vi "06. Native MQTT System.vi"() -> ()   [LabVIEW 2019]
uses:
  Actor/Request -- cluster.ctl
  <vilib>/LabVIEW Open Source Project/MQTT Control Packets/Control Packets/ControlPacket/ControlPacket.lvclass/ControlPacket.ctl
  d83398bf-d288-4447-9c56-1851baa950d7.vi
  04c4b1fc-7be5-4a64-96c3-6608f790954d.vi
  6d0c06f0-3ef9-43f7-be9c-84012acbe03f.vi
  e0405e1f-2754-44b6-a86d-f374eef61912.vi
  <vilib>/LabVIEW Open Source Project/MQTT Control Packets/Control Packets/PUBLISH/PUBLISH.lvclass
  C:/Program Files (x86)/National Instruments/LabVIEW 2019/vi.lib/LabVIEW Open Source Project/MQTT Control Packets/Control Packets/ControlPacket/ControlPacket.lvclass
  <vilib>/JDP Science/JSONtext/JSON text to Variant.vi
  <vilib>/JDP Science/JSONtext/Variant to JSON Text.vi
  <vilib>/JDP Science/JSONtext/LVClass Serializer/JSONtext LVClass Serializer.lvclass
  <vilib>/LabVIEW Open Source Project/MQTT Control Packets/Control Packets/ControlPacket/ControlPacket.lvclass
panel:
  in  "QualifiedName":string="demo/system"
  in  "amplitude":dbl
  in  "Hide Instrument":bool
  in  "Show Instrument":bool
  out "Waveform Chart":dbl(graph)
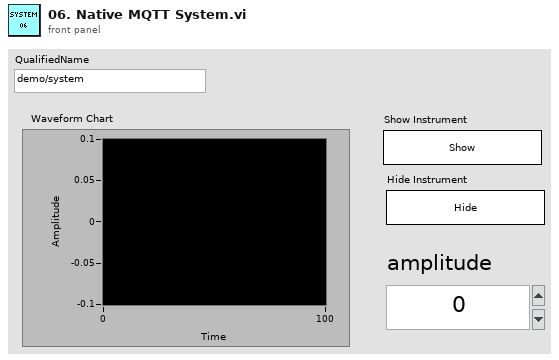
[diagram p1: front panel]
types:
  T1 = typedef "Actor Private Data.ctl" = cluster{"Client":refnum<class "Client.lvclass">, "QualifiedName":string, "EventReg":refnum<event-registration>, "Private Events":T2}
  T2 = typedef "Actor Private Events -- cluster.ctl" = cluster{"Stop":refnum<user-event>, "Subscribe":refnum<user-event>, "Unsubscribe":refnum<user-event>, "publish":refnum<user-event>}
  T3 = typedef "Request -- cluster.ctl" = cluster{"method":string, "<JSON>params":string, "id":string, "reply-topic":string}
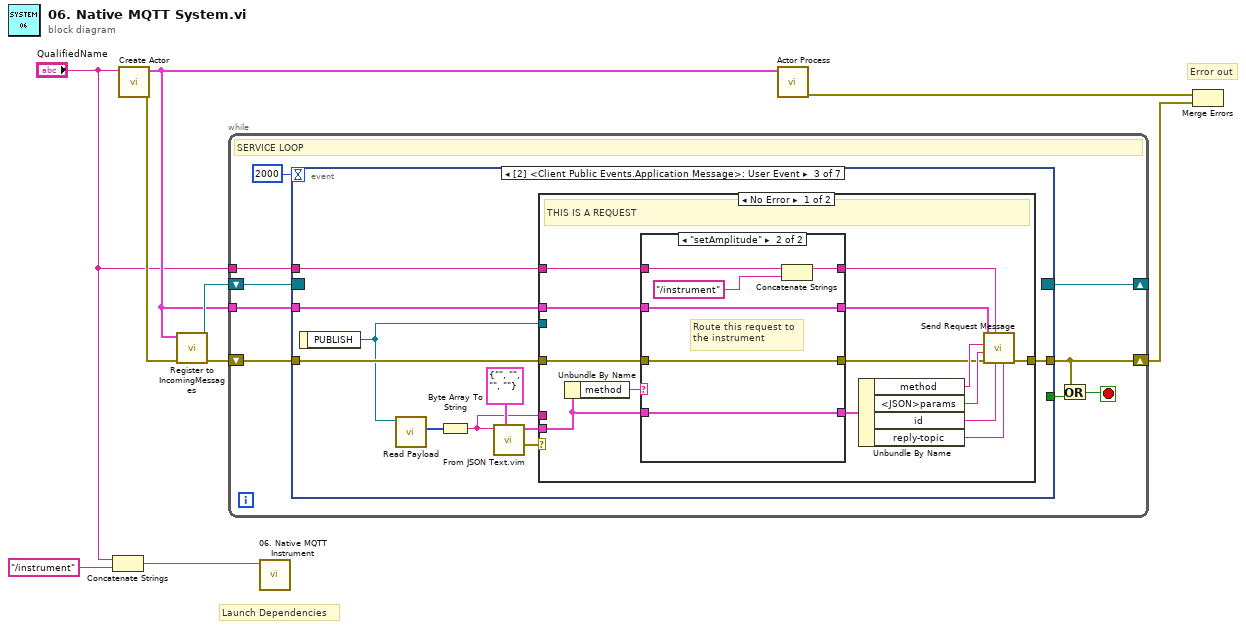
[diagram p0: block diagram]
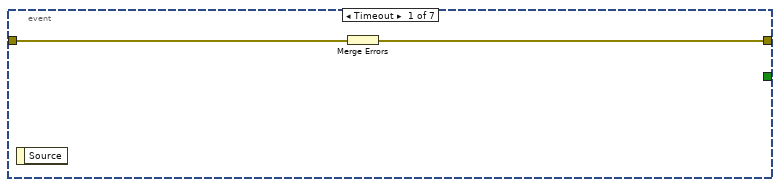
[diagram p2: hidden frame]
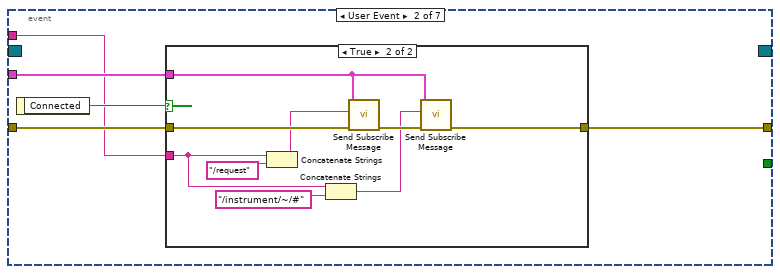
[diagram p3: hidden frame]
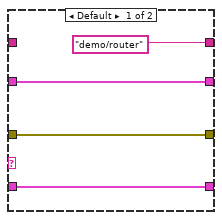
[diagram p5: hidden frame]
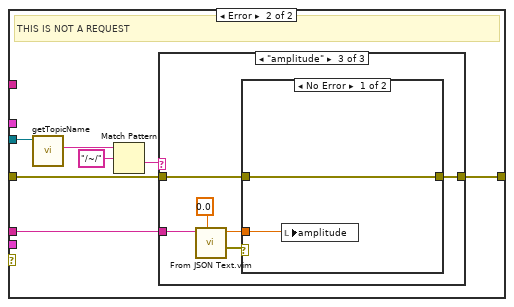
[diagram p6: hidden frame]
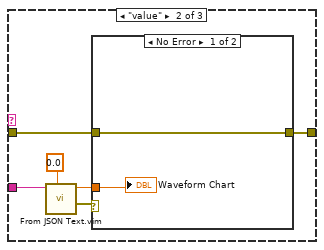
[diagram p8: hidden frame]
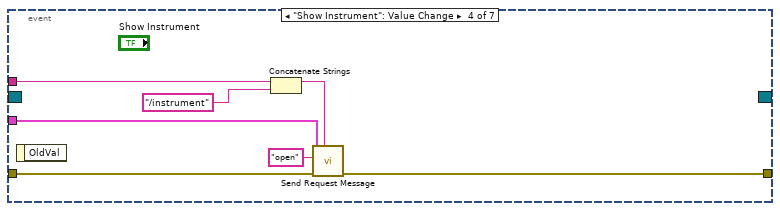
[diagram p11: hidden frame]
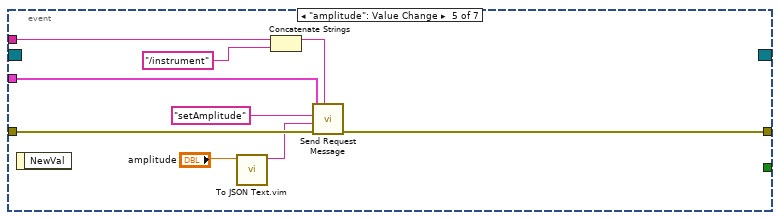
[diagram p12: hidden frame]
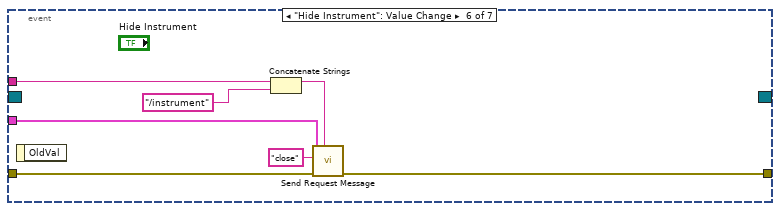
[diagram p13: hidden frame]
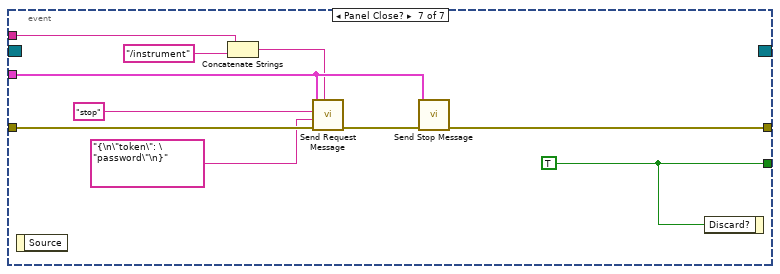
[diagram p14: hidden frame]
diagram:
  # "Launch Dependencies"
  # "Error out"
  n1 = Concatenate Strings("QualifiedName", "/instrument" ("string")) -> (w2:string)
  n2 = call "Create Actor.vi"("QualifiedName"="QualifiedName") -> ("error out"=w8:errorcluster, "Actor Class"=w6:T1)  [unwired: 9 in]
  n3 = call "Register to IncomingMessages.vi"("error in"=w8, "Actor Class"=w6) -> ("error out"=w5:errorcluster, "Incoming Messages"=w7:refnum<event-registration>)  [unwired: 8 in]
  n4 = while {
    tunnel: w6 -> [w16]
    shift-right: [w13] -> _
    shift-left: w7 -> [w14]
    shift-right: [w11] -> w4
    shift-left: w5 -> [w12]
    tunnel: "QualifiedName" -> [w10]
    stop <- w17 stop-if-true
    # "SERVICE LOOP"
    n5 = event shown="[2] <Client Public Events.Application Message>: User Event" {
      selector: w14 -> [_ _ _ _ _ _ _]
      dyn-events: [_ _ _ _ _ _ _] -> w13
      timeout: 2000 -> [_ _ _ _ _ _ _]
      tunnel: [_ _ _ _ _ _ w128] -> w18
      tunnel: w16 -> [_ w23 w41 w99 w108 w115 w124]
      tunnel: [w19 w24 w39 w102 w111 w118 w125] -> w11
      tunnel: w12 -> [w20 w25 w40 w100 w109 w116 w127]
      tunnel: w10 -> [_ w21 w38 w101 w110 w117 w120]
      event Timeout {
        n6 = event-data() -> ()  [unwired: 1 in, 1 out]
        n7 = Merge Errors(w20) -> (w19:errorcluster)
      }
      event User Event {
        n8 = event-data() -> ("Connected"=w22:bool)  [unwired: 1 in]
        n9 = case shown="True" w22 {
          tunnel: w25 -> [w26 w35]
          tunnel: [w26 w28] -> w24
          tunnel: w23 -> [_ w32]
          tunnel: w21 -> [_ w27]
          frame False {
          }
          frame True {
            n10 = Concatenate Strings(w27, "/request" ("QualifiedName")) -> (w30:string)
            n11 = Concatenate Strings(w27, "/instrument/~/#" ("QualifiedName")) -> (w29:string)
            n12 = call "Send Subscribe Message.vi"("error in"=w35, "Topic"=w30, "Actor Class"=w32) -> ("error out"=w33:errorcluster)  [unwired: 8 in]
            n13 = call "Send Subscribe Message.vi"("error in"=w33, "Topic"=w29, "Actor Class"=w32) -> ("error out"=w28:errorcluster)  [unwired: 8 in]
          }
        }
      }
      event User Event {
        n14 = event-data() -> ("PUBLISH"=w37:refnum<class "PUBLISH.lvclass">)  [unwired: 1 in]
        n15 = call <vilib>:"Read Payload.vi"("ControlPacket in"=w37) -> ("Payload"=w45:u8[])  [unwired: 9 in, 1 out]
        n16 = Byte Array To String(unsigned byte array=w45) -> (string=w36:string)
        n17 = call "From JSON Text.vim"("Data Type and Default Value"=T3 {"method"="", "<JSON>params"="", "id"="", "reply-topic"=""} ("request"), "JSON"=w36) -> ("error out"=w43:errorcluster, "Data out"=w42:T3)  [unwired: 8 in]
        n18 = case shown="No Error" w43 {
          tunnel: w42 -> [w52 _]
          tunnel: w41 -> [w51 _]
          tunnel: w40 -> [w50 w72]
          tunnel: [w59 w71] -> w39
          tunnel: w38 -> [w46 _]
          tunnel: w37 -> [_ w74]
          tunnel: w36 -> [_ w70]
          frame No Error {
            # "THIS IS A REQUEST"
            n19 = Unbundle By Name(w52) -> ("method"=w54:string)
            n20 = case shown="\"setAmplitude\"" w54 {
              tunnel: [w63 w69] -> w53
              tunnel: w52 -> [w63 w69]
              tunnel: w51 -> [w61 w67]
              tunnel: w50 -> [w62 w68]
              tunnel: [w62 w68] -> w49
              tunnel: [w61 w67] -> w48
              tunnel: ["demo/router" ("QualifiedName") w65] -> w47
              tunnel: w46 -> [_ w64]
              frame Default {
              }
              frame "setAmplitude" {
                # "Route this request to\nthe instrument"
                n21 = Concatenate Strings(w64, "/instrument" ("string")) -> (w65:string)
              }
            }
            n22 = Unbundle By Name(w53) -> ("method"=w55:string, "<JSON>params"=w58:string, "id"=w57:string, "reply-topic"=w56:string)
            n23 = call "Send Request Message.vi"("reply-topic"=w56, "id"=w57, "Qualified Name"=w47, "error in"=w49, "<JSON>params"=w58, "method"=w55, "Actor Class"=w48) -> ("error out"=w59:errorcluster)  [unwired: 2 in, 2 out]
          }
          frame Error {
            # "THIS IS NOT A REQUEST"
            n24 = call <vilib>:"getTopicName.vi"("PUBLISH in"=w74) -> ("Topic"=w75:string)  [unwired: 8 in, 2 out]
            n25 = Match Pattern(string=w75, regular expression="/~/" ("QualifiedName")) -> (after substring=w73:string)  [unwired: 1 in, 3 out]
            n26 = case shown="\"amplitude\"" w73 {
              tunnel: w72 -> [w77 w79 w88]
              tunnel: [w77 w80 w89] -> w71
              tunnel: w70 -> [_ w83 w92]
              frame Default {
                # "Unhandled packet"
              }
              frame "value" {
                n27 = call "From JSON Text.vim"("Data Type and Default Value"=0.0, "JSON"=w83) -> ("error out"=w81:errorcluster, "Data out"=w78:dbl)  [unwired: 8 in]
                n28 = case shown="No Error" w81 {
                  tunnel: [w85 w86] -> w80
                  tunnel: w79 -> [w85 w86]
                  tunnel: w78 -> [w84 _]
                  frame No Error {
                    "Waveform Chart" <- w84
                  }
                  frame Error {
                    # "invaid packet format"
                  }
                }
              }
              frame "amplitude" {
                n29 = call "From JSON Text.vim"("Data Type and Default Value"=0.0, "JSON"=w92) -> ("error out"=w90:errorcluster, "Data out"=w87:dbl)  [unwired: 8 in]
                n30 = case shown="No Error" w90 {
                  tunnel: [w94 w95] -> w89
                  tunnel: w88 -> [w94 w95]
                  tunnel: w87 -> [w93 _]
                  frame No Error {
                    n31 = local write "amplitude"(w93) -> ()
                  }
                  frame Error {
                    # "invaid packet format"
                  }
                }
              }
            }
          }
        }
      }
      event "Show Instrument": Value Change {
        n32 = event-data() -> ()  [unwired: 1 in, 1 out]
        n33 = Concatenate Strings(w101, "/instrument" ("string")) -> (w98:string)
        n34 = call "Send Request Message.vi"("Qualified Name"=w98, "error in"=w100, "method"="open", "Actor Class"=w99) -> ("error out"=w102:errorcluster)  [unwired: 5 in, 2 out]
      }
      event "amplitude": Value Change {
        n35 = event-data() -> ()  [unwired: 1 in, 1 out]
        n36 = call "To JSON Text.vim"("Anything"="amplitude") -> ("<JSON>"=w103:string)  [unwired: 9 in, 1 out]
        n37 = Concatenate Strings(w110, "/instrument" ("string")) -> (w107:string)
        n38 = call "Send Request Message.vi"("Qualified Name"=w107, "error in"=w109, "<JSON>params"=w103, "method"="setAmplitude", "Actor Class"=w108) -> ("error out"=w111:errorcluster)  [unwired: 4 in, 2 out]
      }
      event "Hide Instrument": Value Change {
        n39 = event-data() -> ()  [unwired: 1 in, 1 out]
        n40 = Concatenate Strings(w117, "/instrument" ("string")) -> (w114:string)
        n41 = call "Send Request Message.vi"("Qualified Name"=w114, "error in"=w116, "method"="close", "Actor Class"=w115) -> ("error out"=w118:errorcluster)  [unwired: 5 in, 2 out]
      }
      event Panel Close? {
        w128 = TRUE ("Discard?")
        n42 = event-data() -> ()  [unwired: 1 in, 1 out]
        n43 = Concatenate Strings(w120, "/instrument" ("string")) -> (w119:string)
        n44 = call "Send Request Message.vi"("Qualified Name"=w119, "error in"=w127, "<JSON>params"="{\n\"token\": \"password\"\n}" ("method"), "method"="stop", "Actor Class"=w124) -> ("error out"=w126:errorcluster)  [unwired: 4 in, 2 out]
        n45 = call "Send Stop Message.vi"("error in"=w126, "Actor Class"=w124) -> ("error out"=w125:errorcluster)  [unwired: 9 in]
        n46 = event-data("Discard?"=w128) -> ()  [unwired: 1 in, 1 out]
      }
    }
    n47 = Or(x=w11, y=w18) -> (x .or. y?=w17:bool)
  }
  n48 = call "06. Native MQTT Instrument.vi"("QualifiedName"=w2) -> ()  [unwired: 11 in]
  n49 = call "Actor Process.vi"("Actor Class"=w6) -> ("error out"=w9:errorcluster)  [unwired: 10 in]
  n50 = Merge Errors(w9, w4) -> ()  [unwired: 1 out]
